vi "Select Units.vi"() -> (0 "Element":string, 1 "Cancelled":bool)   [LabVIEW 2023]
panel:
  in  "Cancel":bool
  in  "OK":bool
  in  "Unit Type":T1(ring)
  in  "Select":i32(listbox)
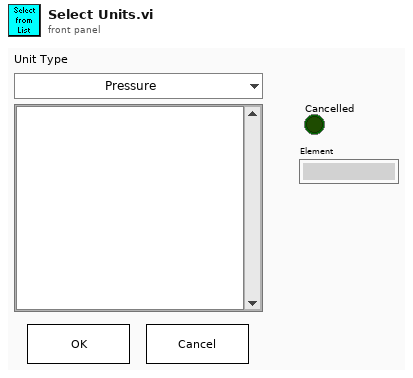
[diagram p1: front panel]
types:
  T1 = enum16{"Pressure", "Force", "Torque", "Distance", "Flow", "Angle", "Angular Velocity", "Acceleration", "Temperature", "Speed", "Voltage", "Current"}
  T2 = cluster{"Unit Section Names":string[], "Section":cluster{"Unit Key Names":string[], "Conversion Table":cluster{"Span":dbl, "Zero":dbl}[][]}[]}
  T3 = cluster{"Unit Key Names":string[], "Conversion Table":cluster{"Span":dbl, "Zero":dbl}[][]}[]
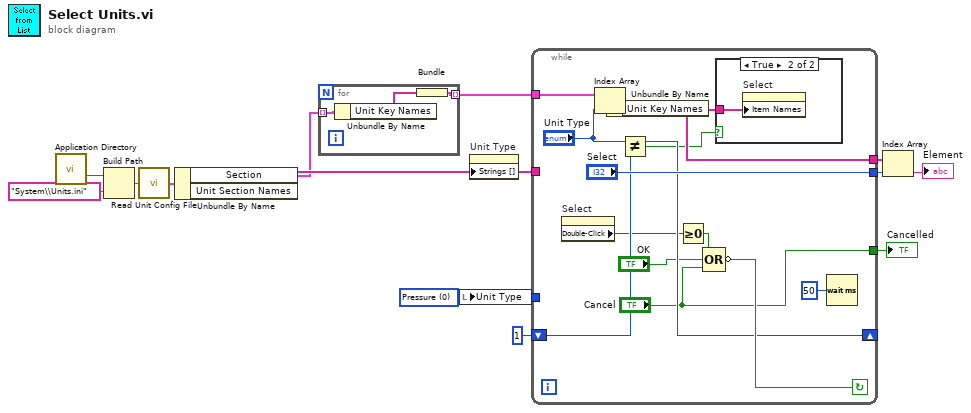
[diagram p0: block diagram]
diagram:
  w9 = u16 0 items=["Pressure", "Force", "Torque", "Distance", "Flow", "Angle", "Angular Velocity", "Acceleration", "Temperature", "Speed", "Voltage", "Current"] ("Unit Type")
  n1 = call <vilib>:"Application Directory.vi"() -> ("Application Directory"=w1:path)
  n2 = Build Path(base path=w1, name or relative path="System\\Units.ini") -> (appended path=w6:path)
  n3 = call "Read Unit Config File.vi"("Unit Config File Path"=w6) -> ("Unit Config File"=w7:T2)
  n4 = Unbundle By Name(w7) -> ("Section"=w2:T3, "Unit Section Names"=w3:string[])
  n5 = for {
    tunnel: w2 -> [w16] mode=indexing
    tunnel: [w14] -> w4 mode=indexing
    n6 = Unbundle By Name(w16) -> ("Unit Key Names"=w15:string[])
    n7 = Bundle("Unit Key Names"=w15) -> (w14:cluster{"Unit Key Names":string[]})  [unwired: 1 in]
  }
  n8 = local write "Unit Type"(w9) -> ()
  n9 = property on="Unit Type" class="Enum (strict)"("Strings []"=w3) -> ()  [unwired: 2 in, 2 out]
  n10 = while {
    tunnel: w9 -> [_]
    tunnel: w4 -> [w23]
    shift-left: u16 1 ("Unit Type") -> [w22]
    shift-right: ["Unit Type"] -> _
    tunnel: [w24] -> w10
    tunnel: w3 -> [_]
    tunnel: ["Select"] -> w12
    tunnel: ["Cancel"] -> w13
    stop <- w28 continue-if-true
    n11 = property on="Select" class="LstBox (strict)"() -> ("Double-Click"=w19:i32)  [unwired: 2 in, 2 out]
    n12 = Index Array(array=w23, index="Unit Type") -> (element=w25:cluster{"Unit Key Names":string[]})
    n13 = Unbundle By Name(w25) -> ("Unit Key Names"=w24:string[])
    n14 = Not Equal?(x="Unit Type", y=w22) -> (x != y?=w20:bool)
    n15 = Greater Or Equal To 0?(x=w19) -> (x >= 0?=w29:bool)
    n16 = Compound Arithmetic op=OR(w29, "OK", "Cancel") -> (invert w28:bool)
    n17 = case shown="True" w20 {
      tunnel: w24 -> [_ w30]
      frame False {
      }
      frame True {
        n18 = property on="Select" class="LstBox (strict)"("Item Names"=w30) -> ()  [unwired: 2 in, 2 out]
      }
    }
    n19 = Wait (ms)(milliseconds to wait=u32 50) -> ()  [unwired: 1 out]
  }
  "Cancelled" <- w13
  n20 = Index Array(array=w10, index=w12) -> (element=→"Element":string)
